vi "Write Key Value Path.vi"(7 "Section Name":string, 8 "error in (no error)":errorcluster, 9 "Value":path, 10 "Key Name":string, 11 "ODBC-Interface in":refnum<class "ODBC-Interface.lvclass">) -> (0 "error out":errorcluster, 2 "found":bool, 3 "ODBC-Interface out":refnum<class "ODBC-Interface.lvclass">)   [LabVIEW 2014, in "DB-Configuration.lvlib" / "ODBC-Interface.lvclass"]
doc: "Write path key value."
uses:
  ODBC-Interface.lvclass
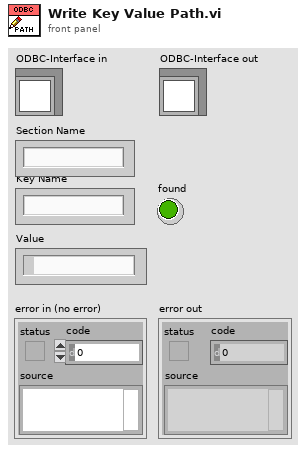
[diagram p1: front panel]
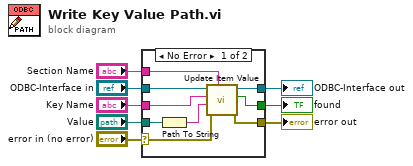
[diagram p0: block diagram]
diagram:
  n1 = case shown="No Error" "error in (no error)" {
    selector: "error in (no error)" -> [w9 w18]
    tunnel: "Section Name" -> [w17 _]
    tunnel: "ODBC-Interface in" -> [w16 w19]
    tunnel: [w15 w19] -> w3
    tunnel: "Key Name" -> [w14 _]
    tunnel: "Value" -> [w13 _]
    tunnel: [w11 w18] -> w1
    tunnel: [w10 _] -> w2
    frame No Error {
      n2 = Path To String(path=w13) -> (string=w12:string)
      n3 = call-dynamic "Update Item Value.vi"("Section Name"=w17, "error in (no error)"=w9, "Value"=w12, "Key Name"=w14, "ODBC-Interface in"=w16) -> ("error out"=w11:errorcluster, "found"=w10:bool, "ODBC-Interface out"=w15:refnum<class "ODBC-Interface.lvclass">)  [unwired: 4 in]
    }
    frame Error {
    }
  }
  "error out" <- w1
  "ODBC-Interface out" <- w3
  "found" <- w2
